vi "Get Parameter Value (array).vi"(10 "Parameter Name":string, 11 "JSON":string) -> (1 "Found":bool, 2 "Parameter Values":string[](array[string]), 3 "Remaining JSON":string)   [LabVIEW 2015, in "NI_Azure_JSON Parsing.lvlib"]
uses:
  NI_Azure_JSON Parsing.lvlib
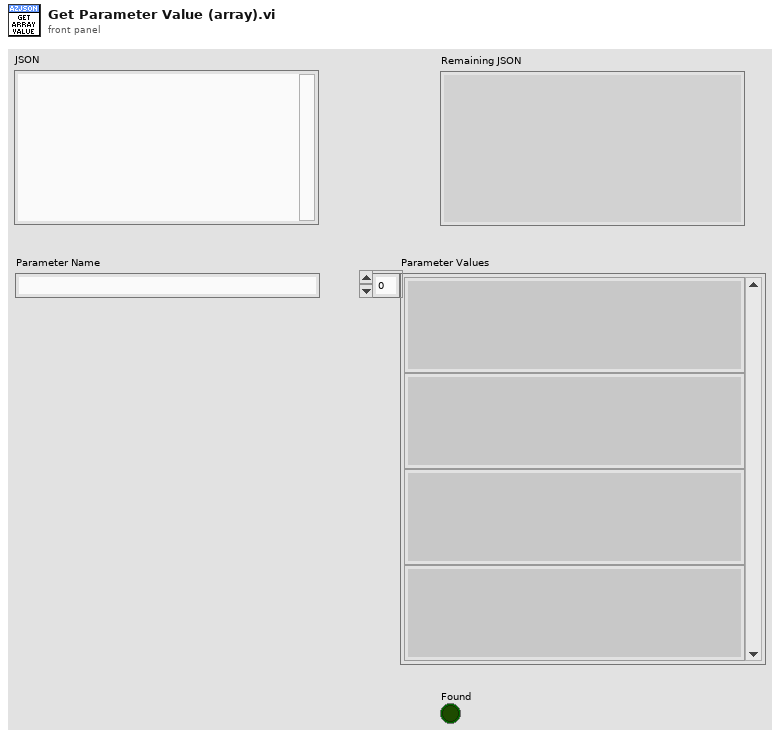
[diagram p1: front panel]
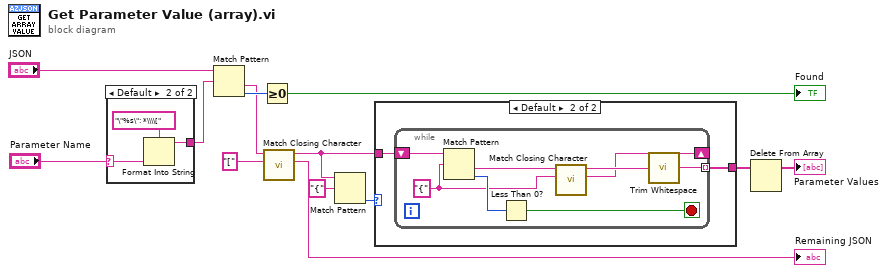
[diagram p0: block diagram]
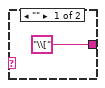
[diagram p2: hidden frame]
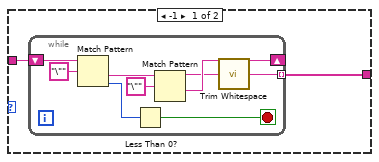
[diagram p3: hidden frame]
diagram:
  n1 = case shown="Default" "Parameter Name" {
    selector: "Parameter Name" -> [_ w17]
    tunnel: ["\\[" w15] -> w9
    frame "" {
    }
    frame Default {
      n2 = Format Into String(format string="\"%s\": *\\\\[", w17) -> (resulting string=w15:string)  [unwired: 2 in, 1 out]
    }
  }
  n3 = Match Pattern(string="JSON", regular expression=w9) -> (after substring=w4:string, offset past match=w8:i32)  [unwired: 1 in, 2 out]
  n4 = Greater Or Equal To 0?(x=w8) -> (x >= 0?=→"Found":bool)
  n5 = call "Match Closing Character.vi"("Open character"="[", "JSON"=w4) -> ("rest of JSON"=→"Remaining JSON":string, "match"=w2:string)  [unwired: 7 in, 1 out]
  n6 = Match Pattern(string=w2, regular expression="{") -> (offset past match=w5:i32)  [unwired: 1 in, 3 out]
  n7 = case shown="Default" w5 {
    tunnel: [w19 w30] -> w13
    tunnel: w2 -> [w18 w29]
    frame -1 {
      n8 = while {
        shift-right: [w23] -> _
        shift-left: w18 -> [w28]
        tunnel: [w20] -> w19 mode=indexing
        stop <- w25 stop-if-true
        n9 = Match Pattern(string=w28, regular expression="\"") -> (after substring=w24:string, offset past match=w26:i32)  [unwired: 1 in, 2 out]
        n10 = Less Than 0?(x=w26) -> (x < 0?=w25:bool)
        n11 = Match Pattern(string=w24, regular expression="\"") -> (before substring=w21:string, after substring=w23:string)  [unwired: 1 in, 2 out]
        n12 = call <vilib>:"Trim Whitespace.vi"("string"=w21) -> ("trimmed string"=w20:string)  [unwired: 1 in]
      }
    }
    frame Default {
      n13 = while {
        shift-right: [w31] -> _
        shift-left: w29 -> [w38]
        tunnel: [w35] -> w30 mode=indexing
        stop <- w36 stop-if-true
        w33 = "{" ("regular expression")
        n14 = Match Pattern(string=w38, regular expression=w33) -> (after substring=w34:string, offset past match=w37:i32)  [unwired: 1 in, 2 out]
        n15 = Less Than 0?(x=w37) -> (x < 0?=w36:bool)
        n16 = call "Match Closing Character.vi"("Open character"=w33, "JSON"=w34) -> ("rest of JSON"=w31:string, "match"=w32:string)  [unwired: 7 in, 1 out]
        n17 = call <vilib>:"Trim Whitespace.vi"("string"=w32) -> ("trimmed string"=w35:string)  [unwired: 1 in]
      }
    }
  }
  n18 = Delete From Array(array=w13) -> (array with subset deleted=→"Parameter Values":string[])  [unwired: 2 in, 1 out]
